vi "midi test.vi"(11 "MIDI file (.mid)":path=path "/home/lvuser/trio.mid") -> (0 "error out":errorcluster, 1 "duration (min:sec)":string="0:00", 2 "note events":dbl[][](array[numeric]), 3 "duration [seconds]":dbl, 4 "Track number: name [channel(s) used]":string="Please select a MIDI file...", 5 "Text":string)   [LabVIEW 2013]
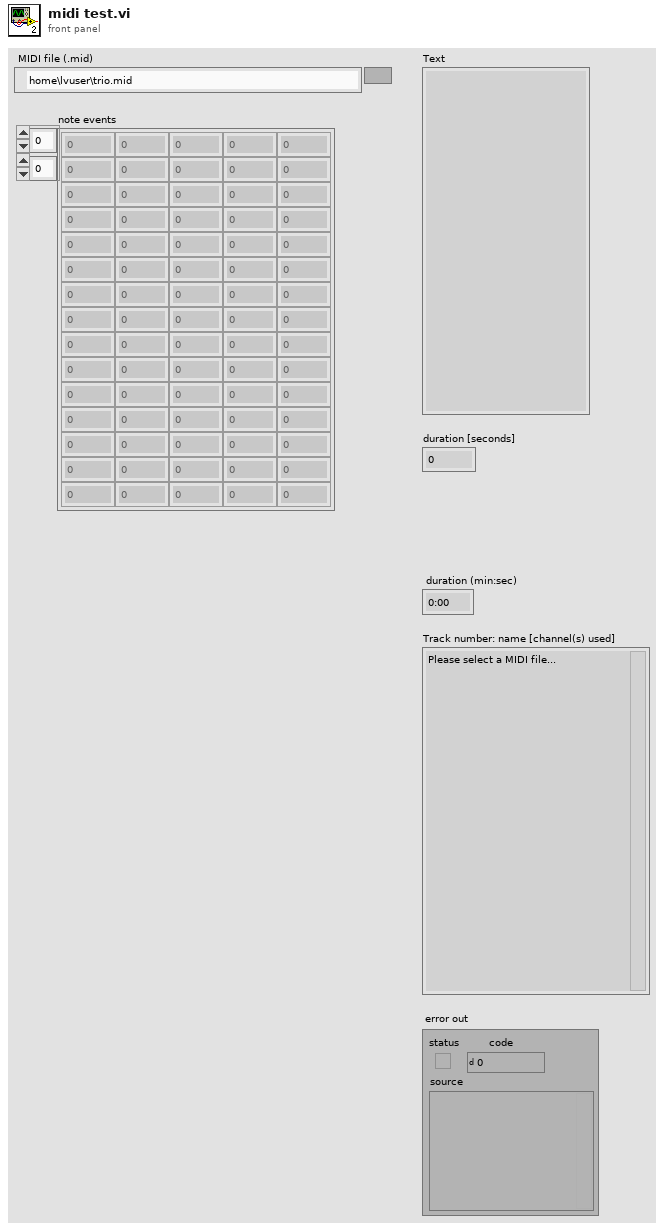
[diagram p1: front panel]
types:
  T1 = cluster{"type":u16, "tracks":u16, "ticks per qnote":u16}
  T2 = cluster{"note events":dbl[][], "duration [seconds]":dbl, "track info":string, "text meta-events":string}
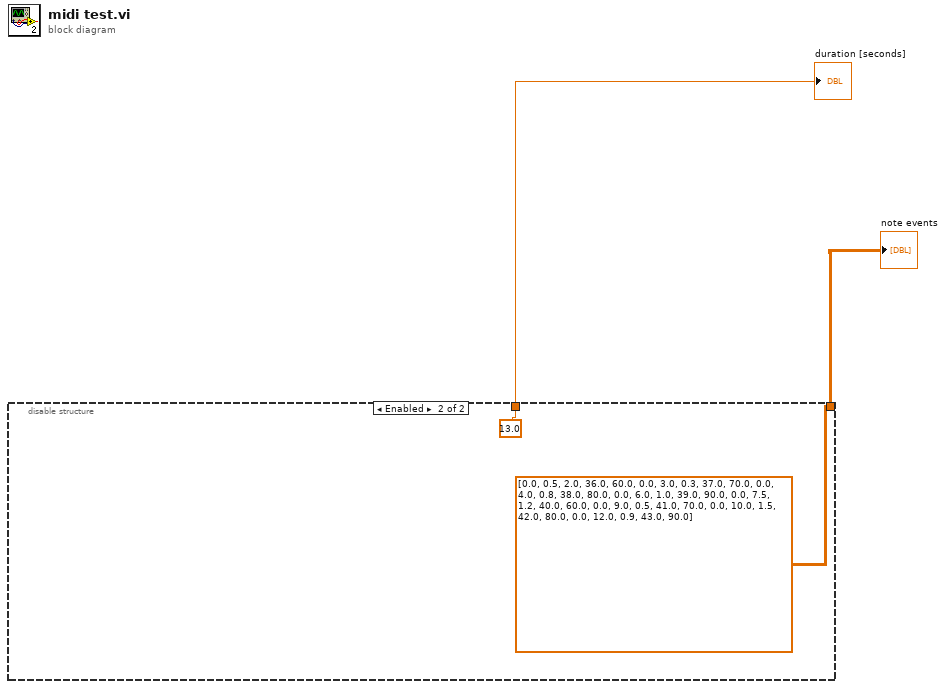
[diagram p0: block diagram]
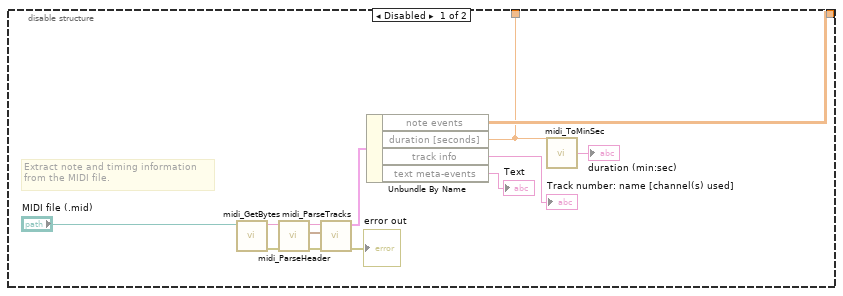
[diagram p2: hidden frame]
diagram:
  n1 = disable-structure shown="Enabled" {
    disable-tunnel: [w3 13.0 ("duration [seconds]")] -> w2
    disable-tunnel: [w4 dbl[][] [[0.0, 0.5, 2.0, 36.0, 60.0], [0.0, 3.0, 0.3, 37.0, 70.0], [0.0, 4.0, 0.8, 38.0, 80.0], [0.0, 6.0, 1.0, 39.0, 90.0], [0.0, 7.5, 1.2, 40.0, 60.0], [0.0, 9.0, 0.5, 41.0, 70.0], [0.0, 10.0, 1.5, 42.0, 80.0], [0.0, 12.0, 0.9, 43.0, 90.0]] ("note events")] -> w1
    frame Disabled {
      # "Extract note and timing information\nfrom the MIDI file."
      n2 = call "midi_GetBytes.vi"("folder name"="MIDI file (.mid)") -> ("error out"=w6:errorcluster, "string"=w13:string)  [unwired: 8 in, 1 out]
      n3 = call "midi_ParseHeader.vi"("error in (no error)"=w6, "string in"=w13) -> ("error out"=w11:errorcluster, "header info"=w7:T1, "string out"=w12:string)  [unwired: 7 in]
      n4 = call "midi_ParseTracks.vi"("error in (no error)"=w11, "header info"=w7, "string in"=w12) -> ("error out"=→"error out":errorcluster, "file contents"=w10:T2)  [unwired: 7 in]
      n5 = Unbundle By Name(w10) -> ("note events"=w4:dbl[][], "duration [seconds]"=w3:dbl, "track info"=→"Track number: name [channel(s) used]":string, "text meta-events"=→"Text":string)
      n6 = call "midi_ToMinSec.vi"("seconds"=w3) -> ("min:sec"=→"duration (min:sec)":string)
    }
    frame Enabled {
    }
  }
  "duration [seconds]" <- w2
  "note events" <- w1
